vi "IDS Camera Engine.vi"(0 "IDS Notifier Name":string="Not a Name", 11 "Camera ID":string[](array[string])) -> ()   [LabVIEW 2020]
uses:
  IDS Controls/IDS Parameters.ctl
  IDS Controls/IDS Parameter List.ctl
  IDS Controls/IDS ROI.ctl
  IDS Controls/IDS Actions.ctl
  IDS Controls/IDS Notifier Element.ctl
  <vilib>/vision/Image Controls.llb/IMAQ Image.ctl
  C:/Users/Photonics03/Documents/Microscope-Control/Device Library/Cameras/IDS/IDS LabView Examples/LabVIEW/ueye.NET/uEyeDotNet.dll
  IDS LabView Examples/LabVIEW/ueye.NET/uEyeDotNet.dll
  Camera Controls/Camera IMAQ Key Info.ctl
panel:
  out "Image Key Error":errorcluster
  out "Frame":u32
  in  "Init Camera":bool
  in  "Quit":bool
  in  "Use Display Module":bool
  in  "Capture":bool
  in  "Live Preview":bool
  in  "Get ROI":bool
  in  "Set ROI":bool
  in  "Get Parameter":bool
  in  "Set Parameter":bool
  in  "File Save Path":path
  in  "# of Frames":u32
  in  "ROI Setup":T1
  in  "IDS Parameter":T2
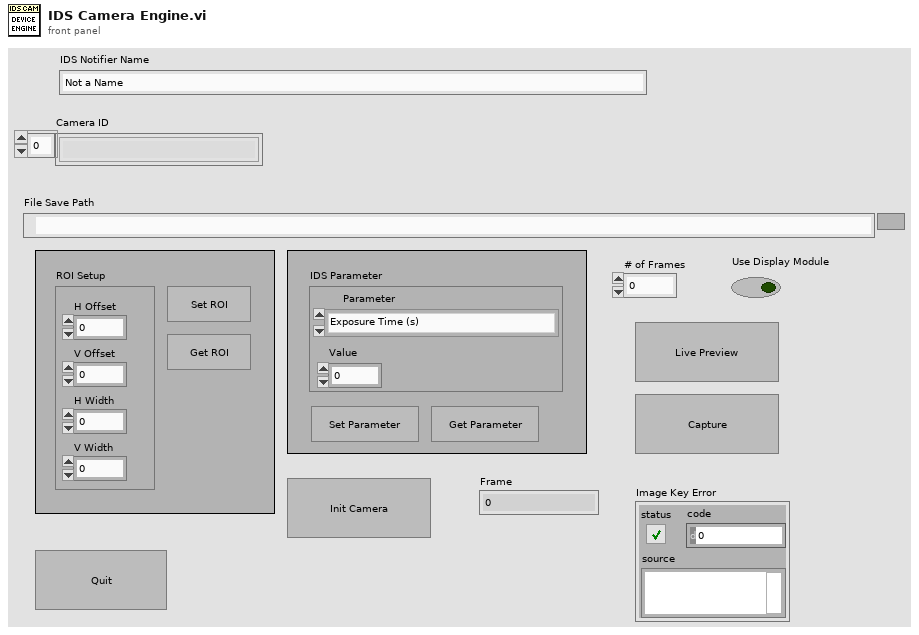
[diagram p1: front panel]
types:
  T1 = typedef "IDS ROI.ctl" = cluster{"H Offset":i32, "V Offset":i32, "H Width":i32, "V Width":i32}
  T2 = typedef "IDS Parameters.ctl" = cluster{"Parameter":T3, "Value":dbl}
  T3 = typedef "IDS Parameter List.ctl" = enum16{"Exposure Time (s)", "Binning"}
  T4 = typedef "IDS Notifier Element.ctl" = cluster{"IDS Actions":T5, "Received?":bool, "IDS Parameter":T2, "IDS ROI":T1, "Running?":bool, "File Path":path, "# of frames":u32, "Image Ref":T6, "Error":errorcluster, "Binning":i32}
  T5 = typedef "IDS Actions.ctl" = enum16{"Error Check", "Initialize", "Preview", "Record", "Abort", "Record Settings", "Set Parameter", "Get Parameter", "Set ROI", "Get ROI", "Status", "Quit"}
  T6 = typedef "IMAQ Image.ctl" = refnum<image>
  T7 = typedef "Image Type" = u32
  T8 = typedef "Camera IMAQ Key Info.ctl" = cluster{"Frame":u32, "Sensor Height":i32, "Sensor Width":i32, "ROI Height":i32, "ROI Width":i32, "ROI Enable?":bool, "Bit per Pixel":u8}
  T9 = enum32{"Invalid", "Standard", "Closed", "Hidden", "Minimized", "Maximized"}
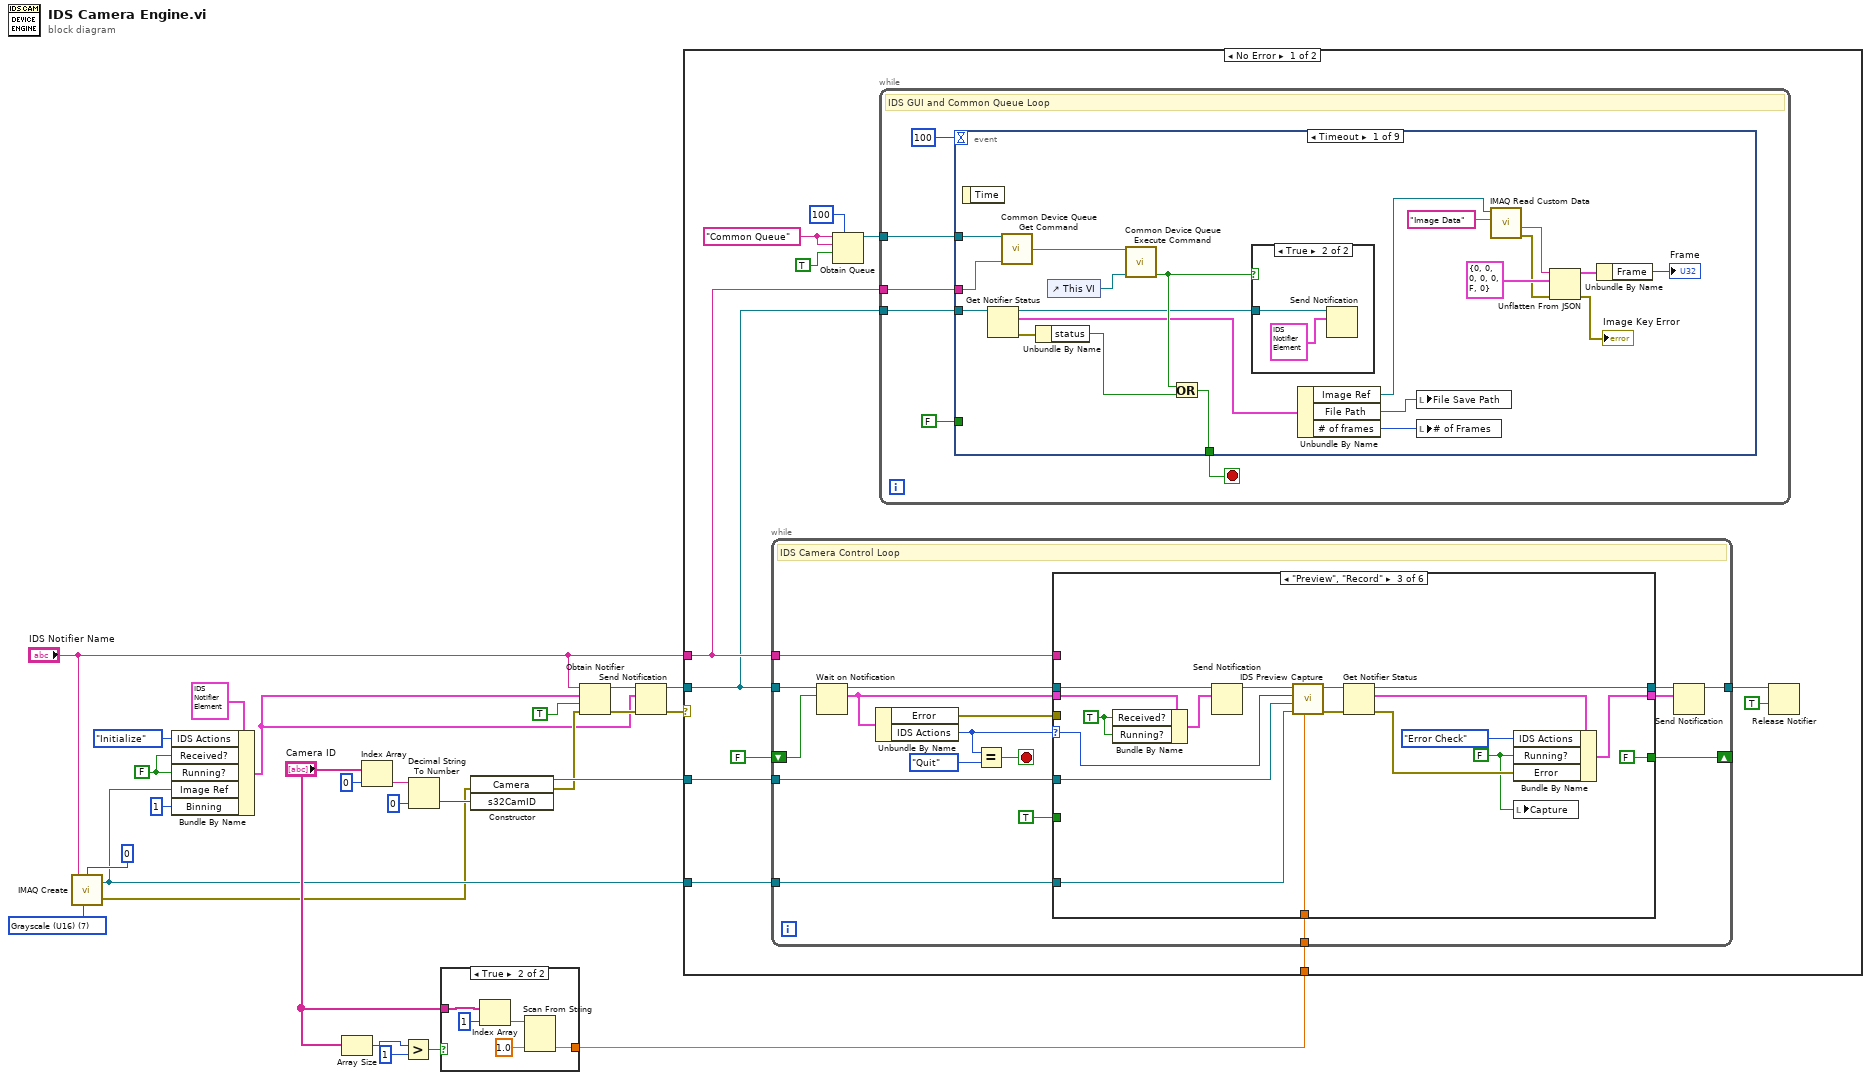
[diagram p0: block diagram]
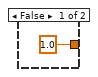
[diagram p2: hidden frame]
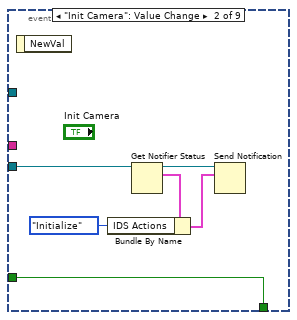
[diagram p4: hidden frame]
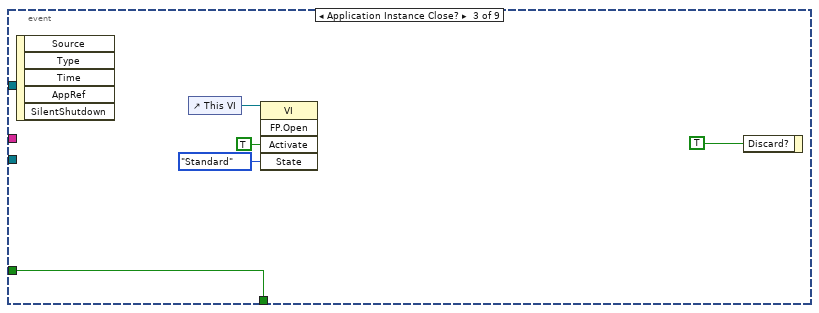
[diagram p5: hidden frame]
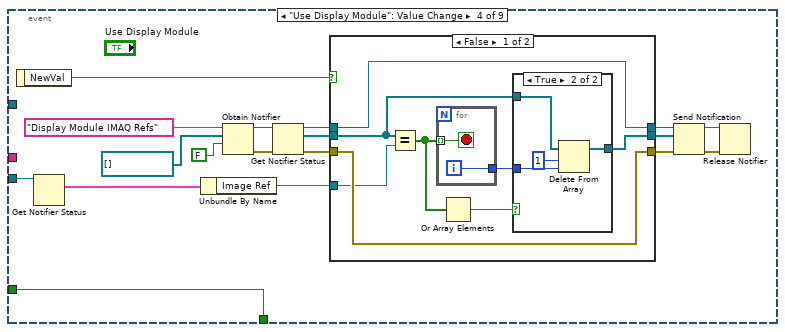
[diagram p6: hidden frame]
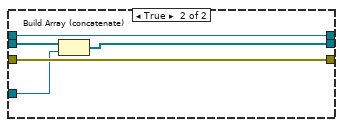
[diagram p8: hidden frame]
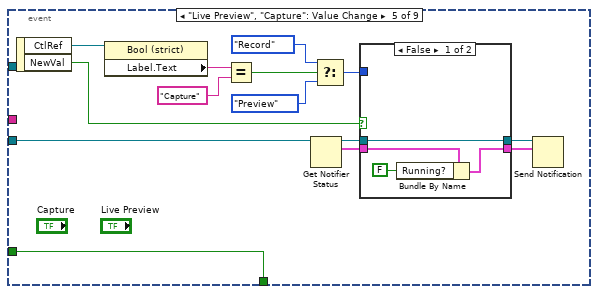
[diagram p9: hidden frame]
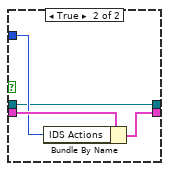
[diagram p10: hidden frame]
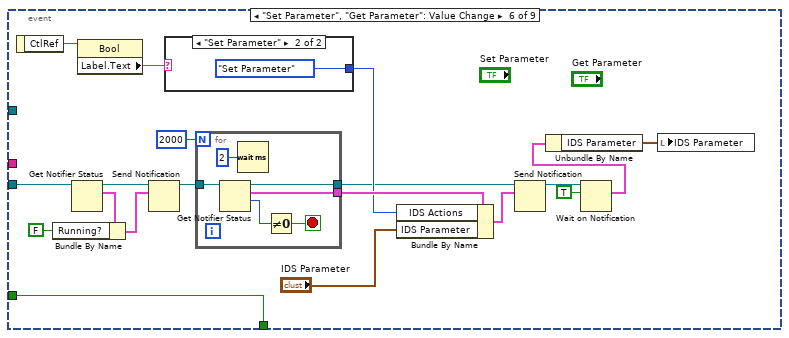
[diagram p11: hidden frame]
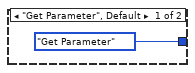
[diagram p12: hidden frame]
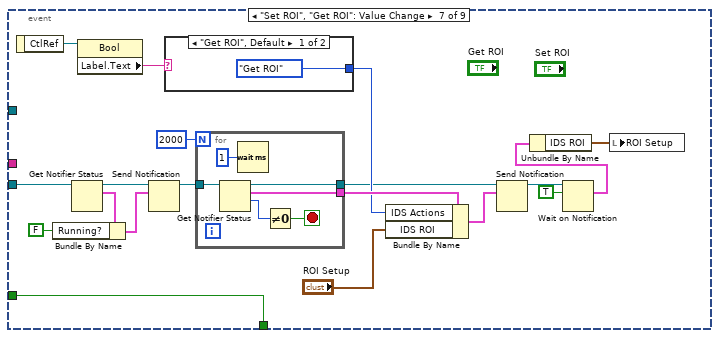
[diagram p13: hidden frame]
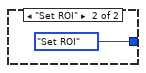
[diagram p14: hidden frame]
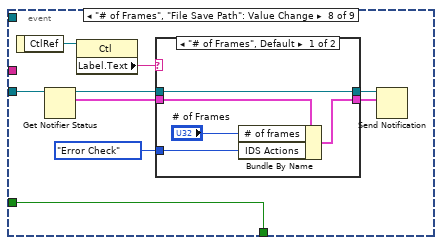
[diagram p15: hidden frame]
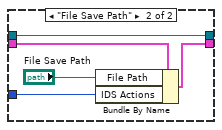
[diagram p16: hidden frame]
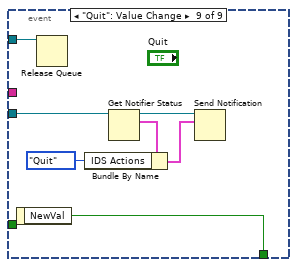
[diagram p17: hidden frame]
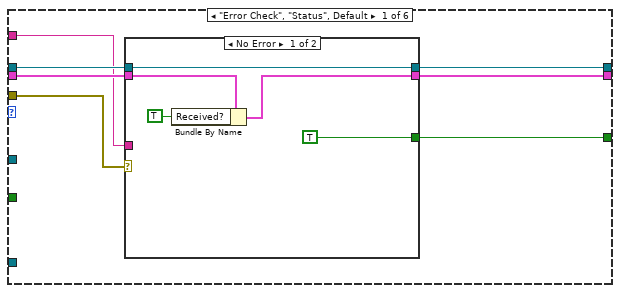
[diagram p18: hidden frame]
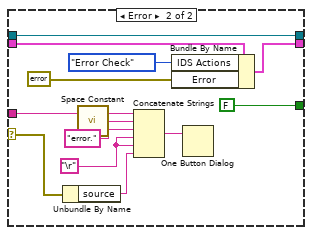
[diagram p19: hidden frame]
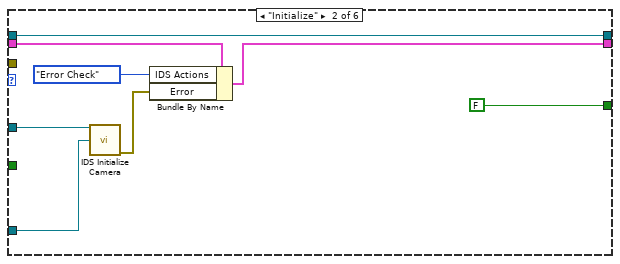
[diagram p20: hidden frame]
diagram:
  w2 = FALSE ("Received?")
  w16 = T7 7 items=["Grayscale (U8)", "Grayscale (I16)", "Grayscale (SGL)", "Complex (CSG)", "RGB (U32)", "HSL (U32)", "RGB (U64)", "Grayscale (U16)"] ("Image Type")
  n1 = call "IMAQ Create"("Border Size"=0, "Image Name"="IDS Notifier Name", "Image Type"=w16) -> ("New Image"=w14:T6, "error out"=w6:errorcluster)  [unwired: 2 in]
  n2 = Bundle By Name(cluster=T4 {"IDS Actions"=enum."Initialize", "Received?"=FALSE, "IDS Parameter"={"Parameter"=enum."Exposure Time (s)", "Value"=0.0}, "IDS ROI"={"H Offset"=0, "V Offset"=0, "H Width"=0, "V Width"=0}, "Running?"=FALSE, "File Path"=path "", "# of frames"=0, "Image Ref"=refnum, "Error"={"status"=FALSE, "code"=0, "source"=""}, "Binning"=0} ("IDS Camera Cluster"), "IDS Actions"=IDS_Actions."Initialize", "Received?"=w2, "Running?"=w2, "Image Ref"=w14, "Binning"=1) -> (w5:T4)
  n3 = Array Size(array="Camera ID") -> (size(s)=w12:i32)
  n4 = Index Array(array="Camera ID", index=0) -> (element=w19:string)
  n5 = Greater?(x=w12, y=1) -> (0:w11:bool)
  n6 = Decimal String To Number(string=w19, default (0L)=0 ("default (0 I32)")) -> (number=w7:i32)  [unwired: 1 in, 1 out]
  n7 = case shown="True" w11 {
    tunnel: "Camera ID" -> [_ w30]
    tunnel: [1.0 ("default (0 dbl)") w32] -> w13
    frame False {
    }
    frame True {
      n8 = Index Array(array=w30, index=1) -> (element=w31:string)
      n9 = Scan From String(input string=w31, default 1=1.0 ("default (0 dbl)")) -> (output 1=w32:dbl)  [unwired: 3 in, 3 out]
    }
  }
  n10 = constructor class="Camera"(error in=w6, "s32CamID"=w7) -> (reference out=w9:refnum<k24>, error out=w8:errorcluster)  [unwired: 2 in, 2 out]
  n11 = Obtain Notifier(name (unnamed)="IDS Notifier Name", notification data type=w5, create if not found? (T)=TRUE, error in (no error)=w8) -> (notifier out=w25:refnum<notifier>, error out=w24:errorcluster)  [unwired: 1 out]
  n12 = Send Notification(notification=w5, notifier=w25, error in (no error)=w24) -> (notifier out=w23:refnum<notifier>, error out=w22:errorcluster)
  n13 = case shown="No Error" w22 {
    selector: w22 -> [_ w341]
    tunnel: w23 -> [w34 w342]
    tunnel: "IDS Notifier Name" -> [w35 w340]
    tunnel: w9 -> [w42 w333]
    tunnel: w14 -> [w41 w332]
    tunnel: w13 -> [w33 _]
    frame No Error {
      w39 = "Common Queue" ("Unique Notifier Name")
      n14 = while {
        tunnel: w34 -> [w239]
        tunnel: [w240] -> w43
        tunnel: w42 -> [w233]
        tunnel: w41 -> [w232]
        shift-right: [w229] -> _
        shift-left: FALSE -> [w231]
        tunnel: w35 -> [w227]
        tunnel: w33 -> [w225]
        stop <- w241 stop-if-true
        # "IDS Camera Control Loop"
        n15 = Wait on Notification(notifier=w239, ignore previous (F)=w231) -> (notifier out=w238:refnum<notifier>, notification=w237:T4)  [unwired: 2 in, 2 out]
        n16 = Unbundle By Name(w237) -> ("Error"=w226:errorcluster, "IDS Actions"=w236:T5)
        n17 = Equal?(x=w236, y=IDS_Actions."Quit") -> (x = y?=w241:bool)
        n18 = case shown="\"Preview\", \"Record\"" w236 {
          selector: w236 -> [_ _ w277 w298 w312 _]
          tunnel: w238 -> [w247 w274 w292 w294 w315 w327]
          tunnel: [w246 w274 w289 w303 w306 w327] -> w234
          tunnel: w237 -> [w245 w272 w291 _ _ w325]
          tunnel: w227 -> [w244 _ _ _ _ _]
          tunnel: w233 -> [_ w273 w278 w297 w314 w321]
          tunnel: w232 -> [_ w267 w279 _ w313 w319]
          tunnel: [w243 w269 w288 w299 w305 w323] -> w230
          tunnel: [w248 FALSE FALSE FALSE w316 w326] -> w229
          tunnel: TRUE -> [_ _ _ _ w316 w326]
          tunnel: w226 -> [w242 _ _ w296 _ w317]
          tunnel: w225 -> [_ _ w275 _ _ _]
          frame "Error Check", "Status", Default {
            n19 = case shown="No Error" w242 {
              selector: w242 -> [_ w256]
              tunnel: w245 -> [w251 w266]
              tunnel: [TRUE FALSE] -> w248
              tunnel: [w253 w263] -> w246
              tunnel: w247 -> [w253 w263]
              tunnel: w244 -> [_ w262]
              tunnel: [w249 w258] -> w243
              frame No Error {
                n20 = Bundle By Name(cluster=w251, "Received?"=TRUE) -> (w249:T4)
              }
              frame Error {
                w257 = "\r"
                n21 = Unbundle By Name(w256) -> ("source"=w255:string)
                n22 = call <vilib>:"Space Constant.vi"() -> ("String"=w261:string)
                n23 = Concatenate Strings(w262, w261, "error." ("string"), w257, w257, w255) -> (w259:string)
                n24 = Bundle By Name(cluster=w266, "IDS Actions"=IDS_Actions."Error Check", "Error"=errorcluster {"status"=FALSE, "code"=0, "source"=""}) -> (w258:T4)
                n25 = One Button Dialog(message=w259) -> ()  [unwired: 1 in, 1 out]
              }
            }
          }
          frame "Initialize" {
            n26 = call "IDS Initialize Camera.vi"("Camera ID"=w273, "IDS Cam Img Ref"=w267) -> ("Error Out"=w270:errorcluster)  [unwired: 12 in, 1 out]
            n27 = Bundle By Name(cluster=w272, "IDS Actions"=IDS_Actions."Error Check", "Error"=w270) -> (w269:T4)
          }
          frame "Preview", "Record" {
            w276 = FALSE ("Running?")
            w285 = TRUE ("Received?")
            n28 = Bundle By Name(cluster=w291, "Received?"=w285, "Running?"=w285) -> (w287:T4)
            n29 = Send Notification(notification=w287, notifier=w292) -> (notifier out=w284:refnum<notifier>)  [unwired: 1 in, 1 out]
            n30 = call "IDS Preview Capture.vi"("Pixel Size (µm)"=w275, "Image Ref"=w279, "IDS Camera Ref"=w278, "IDS Actions"=w277, "IDS Notifier"=w284) -> ("Error"=w281:errorcluster, "IDS Notifier"=w283:refnum<notifier>)  [unwired: 5 in]
            n31 = Get Notifier Status(notifier=w283, error in (no error)=w281) -> (notifier out=w289:refnum<notifier>, current notification=w282:T4, error out=w280:errorcluster)  [unwired: 2 out]
            n32 = Bundle By Name(cluster=w282, "IDS Actions"=IDS_Actions."Error Check", "Running?"=w276, "Error"=w280) -> (w288:T4)
            n33 = local write "Capture"(w276) -> ()
          }
          frame "Set Parameter", "Get Parameter" {
            n34 = call "IDS Set Get Parameter.vi"("IDS Notifier"=w294, "IDS Actions"=w298, "IDS Camera Ref"=w297, "Error"=w296) -> ("IDS Notifier"=w304:refnum<notifier>, "Error"=w300:errorcluster)  [unwired: 10 in]
            n35 = Get Notifier Status(notifier=w304) -> (notifier out=w303:refnum<notifier>, current notification=w302:T4)  [unwired: 1 in, 3 out]
            n36 = Bundle By Name(cluster=w302, "IDS Actions"=IDS_Actions."Error Check", "Error"=w300, "Received?"=TRUE) -> (w299:T4)
          }
          frame "Set ROI", "Get ROI" {
            n37 = call "IDS Set Get ROI.vi"("IDS Notifier Ref"=w315, "IDS Actions"=w312, "IDS Camera Ref"=w314, "IDS Image Ref"=w313) -> ("IDS Notifier Ref (Dup)"=w307:refnum<notifier>, "Error"=w308:errorcluster)  [unwired: 10 in]
            n38 = Get Notifier Status(notifier=w307) -> (notifier out=w306:refnum<notifier>, current notification=w311:T4)  [unwired: 1 in, 3 out]
            n39 = Bundle By Name(cluster=w311, "IDS Actions"=IDS_Actions."Error Check", "Error"=w308, "Received?"=TRUE) -> (w305:T4)
          }
          frame "Quit" {
            n40 = call "IMAQ Dispose"("Image"=w319) -> ()  [unwired: 5 in, 1 out]
            n41 = invoke class="Camera" method="Exit"(reference=w321, error in=w317) -> (reference out=w322:refnum<k24>, error out=w320:errorcluster)  [unwired: 1 in, 1 out]
            n42 = Close Reference(reference=w322, error in (no error)=w320) -> (error out=w318:errorcluster)
            n43 = Bundle By Name(cluster=w325, "Received?"=TRUE, "Error"=w318) -> (w323:T4)
          }
        }
        n44 = Send Notification(notification=w230, notifier=w234) -> (notifier out=w240:refnum<notifier>)  [unwired: 1 in, 1 out]
      }
      n45 = Obtain Queue(max queue size (-1, unlimited)=100, name (unnamed)=w39, element data type=w39, create if not found? (T)=TRUE) -> (queue out=w36:refnum<queue>)  [unwired: 1 in, 2 out]
      n46 = while {
        tunnel: w36 -> [w49]
        tunnel: w35 -> [w47]
        tunnel: w34 -> [w48]
        stop <- w46 stop-if-true
        # "IDS GUI and Common Queue Loop"
        n47 = event shown="[0] Timeout" {
          selector: _ -> [_ _ _ _ _ _ _ _ _]
          dyn-events: _ -> [_ _ _ _ _ _ _ _ _]
          timeout: 100 -> [_ _ _ _ _ _ _ _ _]
          tunnel: w49 -> [w65 _ _ _ _ _ _ _ w224]
          tunnel: w48 -> [w64 w78 _ w102 w127 w161 w188 w205 w223]
          tunnel: w47 -> [w63 _ _ _ _ _ _ _ _]
          tunnel: [w62 w79 w84 w85 w136 w163 w190 w207 w218] -> w46
          tunnel: FALSE -> [_ w79 w84 w85 w136 w163 w190 w207 _]
          event Timeout {
            n48 = event-data() -> ()  [unwired: 1 in, 1 out]
            n49 = Get Notifier Status(notifier=w64) -> (notifier out=w66:refnum<notifier>, current notification=w59:T4, error out=w71:errorcluster)  [unwired: 1 in, 2 out]
            n50 = call "Common Device Queue Get Command.vi"("Common Queue"=w65, "Notifier Name"=w63) -> ("Command"=w70:string)  [unwired: 12 in, 1 out]
            n51 = Unbundle By Name(w71) -> ("status"=w68:bool)
            n52 = control-ref of="This VI"() -> (w69:refnum<vi>)
            n53 = call "Common Device Queue Execute Command.vi"("Common Command"=w70, "VI Refnum"=w69) -> ("Quit?"=w67:bool)  [unwired: 12 in, 1 out]
            n54 = Or(x=w67, y=w68) -> (x .or. y?=w62:bool)
            n55 = case shown="True" w67 {
              tunnel: w66 -> [_ w73]
              frame False {
              }
              frame True {
                n56 = Send Notification(notification=T4 {"IDS Actions"=enum."Quit", "Received?"=FALSE, "IDS Parameter"={"Parameter"=enum."Exposure Time (s)", "Value"=0.0}, "IDS ROI"={"H Offset"=0, "V Offset"=0, "H Width"=0, "V Width"=0}, "Running?"=FALSE, "File Path"=path "", "# of frames"=0, "Image Ref"=refnum, "Error"={"status"=FALSE, "code"=0, "source"=""}, "Binning"=0} ("IDS Camera Cluster"), notifier=w73) -> ()  [unwired: 1 in, 2 out]
              }
            }
            n57 = Unbundle By Name(w59) -> ("Image Ref"=w57:T6, "File Path"=w61:path, "# of frames"=w60:u32)
            n58 = local write "File Save Path"(w61) -> ()
            n59 = local write "# of Frames"(w60) -> ()
            n60 = call "IMAQ Read Custom Data"("Key"="Image Data", "Image"=w57) -> ("error out"=w52:errorcluster, "Custom Data Out"=w55:string)  [unwired: 7 in, 1 out]
            n61 = Unflatten From JSON(JSON string=w55, type and defaults=T8 {"Frame"=0, "Sensor Height"=0, "Sensor Width"=0, "ROI Height"=0, "ROI Width"=0, "ROI Enable?"=FALSE, "Bit per Pixel"=0} ("Camera IMAQ Key Info"), error in (no error)=w52) -> (value=w54:T8, error out=→"Image Key Error":errorcluster)  [unwired: 4 in]
            n62 = Unbundle By Name(w54) -> ("Frame"=→"Frame":u32)
          }
          event "Init Camera": Value Change {
            n63 = event-data() -> ()  [unwired: 1 in, 1 out]
            n64 = Get Notifier Status(notifier=w78) -> (notifier out=w74:refnum<notifier>, current notification=w77:T4)  [unwired: 1 in, 3 out]
            n65 = Bundle By Name(cluster=w77, "IDS Actions"=IDS_Actions."Initialize") -> (w75:T4)
            n66 = Send Notification(notification=w75, notifier=w74) -> ()  [unwired: 1 in, 2 out]
          }
          event Application Instance Close? {
            n67 = event-data() -> ()  [unwired: 1 in, 5 out]
            n68 = control-ref of="This VI"() -> (w81:refnum<vi>)
            n69 = invoke class="VI" method="FP.Open"(reference=w81, "Activate"=TRUE ("Activate?"), "State"=T9."Standard") -> ()  [unwired: 2 in, 5 out]
            n70 = event-data("Discard?"=TRUE) -> ()  [unwired: 1 in, 1 out]
          }
          event "Use Display Module": Value Change {
            n71 = event-data() -> ("NewVal"=w87:bool)  [unwired: 1 in]
            n72 = Get Notifier Status(notifier=w102) -> (current notification=w101:T4)  [unwired: 1 in, 4 out]
            n73 = Unbundle By Name(w101) -> ("Image Ref"=w86:T6)
            n74 = Obtain Notifier(name (unnamed)="Display Module IMAQ Refs", notification data type=T6[] [], create if not found? (T)=FALSE) -> (notifier out=w94:refnum<notifier>, error out=w93:errorcluster)  [unwired: 1 in, 1 out]
            n75 = Get Notifier Status(notifier=w94, error in (no error)=w93) -> (notifier out=w95:refnum<notifier>, current notification=w97:T6[], error out=w96:errorcluster)  [unwired: 2 out]
            n76 = case shown="False" w87 {
              tunnel: w95 -> [w110 w120]
              tunnel: w96 -> [w104 w119]
              tunnel: w97 -> [w106 w122]
              tunnel: [w105 w121] -> w100
              tunnel: [w110 w120] -> w98
              tunnel: [w104 w119] -> w99
              tunnel: w86 -> [w103 w118]
              frame False {
                n77 = Equal?(x=w106, y=w103) -> (x = y?=w109:bool[])
                n78 = for {
                  tunnel: w109 -> [w117] mode=indexing
                  tunnel: [w116] -> w107
                  i -> [w116]
                  stop <- w117 stop-if-true
                }
                n79 = Or Array Elements(Boolean array=w109) -> (logical OR=w108:bool)
                n80 = case shown="True" w108 {
                  tunnel: w107 -> [_ w114]
                  tunnel: w106 -> [w111 w113]
                  tunnel: [w111 w112] -> w105
                  frame False {
                  }
                  frame True {
                    n81 = Delete From Array(array=w113, length=1, index=w114) -> (array with subset deleted=w112:T6[])  [unwired: 1 out]
                  }
                }
              }
              frame True {
                n82 = Build Array (concatenate)(w122, w118) -> (w121:T6[])
              }
            }
            n83 = Send Notification(notification=w100, notifier=w98, error in (no error)=w99) -> (notifier out=w92:refnum<notifier>, error out=w91:errorcluster)
            n84 = Release Notifier(notifier=w92, error in (no error)=w91) -> ()  [unwired: 1 in, 3 out]
          }
          event "Live Preview", "Capture": Value Change {
            n85 = event-data() -> ("CtlRef"=w135:refnum<vi>, "NewVal"=w129:bool)  [unwired: 1 in]
            n86 = property class="Bool (strict)"(reference=w135) -> ("Label.Text"=w134:string)  [unwired: 1 in, 2 out]
            n87 = Equal?(x=w134, y="Capture") -> (x = y?=w132:bool)
            n88 = Get Notifier Status(notifier=w127) -> (notifier out=w126:refnum<notifier>, current notification=w125:T4)  [unwired: 1 in, 3 out]
            n89 = Select(t=IDS_Actions."Record" ("y"), s=w132, f=IDS_Actions."Preview" ("y")) -> (s? t:f=w128:T5)
            n90 = case shown="False" w129 {
              tunnel: w128 -> [_ w143]
              tunnel: w126 -> [w138 w142]
              tunnel: w125 -> [w140 w144]
              tunnel: [w138 w142] -> w124
              tunnel: [w137 w141] -> w123
              frame False {
                n91 = Bundle By Name(cluster=w140, "Running?"=FALSE) -> (w137:T4)
              }
              frame True {
                n92 = Bundle By Name(cluster=w144, "IDS Actions"=w143) -> (w141:T4)
              }
            }
            n93 = Send Notification(notification=w123, notifier=w124) -> ()  [unwired: 1 in, 2 out]
          }
          event "Set Parameter", "Get Parameter": Value Change {
            n94 = event-data() -> ("CtlRef"=w162:refnum<vi>)  [unwired: 1 in]
            n95 = Get Notifier Status(notifier=w161) -> (notifier out=w156:refnum<notifier>, current notification=w159:T4)  [unwired: 1 in, 3 out]
            n96 = Bundle By Name(cluster=w159, "Running?"=FALSE) -> (w155:T4)
            n97 = property class="Bool"(reference=w162) -> ("Label.Text"=w160:string)  [unwired: 1 in, 2 out]
            n98 = Send Notification(notification=w155, notifier=w156) -> (notifier out=w154:refnum<notifier>)  [unwired: 1 in, 1 out]
            n99 = case shown="\"Set Parameter\"" w160 {
              tunnel: [IDS_Actions."Get Parameter" ("IDS Actions") IDS_Actions."Set Parameter" ("IDS Actions")] -> w151
              frame "Get Parameter", Default {
              }
              frame "Set Parameter" {
              }
            }
            n100 = for {
              N: 2000 -> [_]
              tunnel: w154 -> [w168]
              tunnel: [w167] -> w150
              tunnel: [w166] -> w153
              stop <- w164 stop-if-true
              n101 = Get Notifier Status(notifier=w168) -> (notifier out=w167:refnum<notifier>, current notification=w166:T4, # waiting=w165:i32)  [unwired: 1 in, 2 out]
              n102 = Wait (ms)(milliseconds to wait=u32 2) -> ()  [unwired: 1 out]
              n103 = Not Equal To 0?(x=w165) -> (x != 0?=w164:bool)
            }
            n104 = Bundle By Name(cluster=w153, "IDS Actions"=w151, "IDS Parameter"="IDS Parameter") -> (w149:T4)
            n105 = Send Notification(notification=w149, notifier=w150) -> (notifier out=w148:refnum<notifier>)  [unwired: 1 in, 1 out]
            n106 = Wait on Notification(notifier=w148, ignore previous (F)=TRUE) -> (notification=w146:T4)  [unwired: 2 in, 3 out]
            n107 = Unbundle By Name(w146) -> ("IDS Parameter"=w145:T2)
            n108 = local write "IDS Parameter"(w145) -> ()
          }
          event "Set ROI", "Get ROI": Value Change {
            n109 = event-data() -> ("CtlRef"=w189:refnum<vi>)  [unwired: 1 in]
            n110 = Get Notifier Status(notifier=w188) -> (notifier out=w183:refnum<notifier>, current notification=w186:T4)  [unwired: 1 in, 3 out]
            n111 = Bundle By Name(cluster=w186, "Running?"=FALSE) -> (w182:T4)
            n112 = property class="Bool"(reference=w189) -> ("Label.Text"=w187:string)  [unwired: 1 in, 2 out]
            n113 = Send Notification(notification=w182, notifier=w183) -> (notifier out=w181:refnum<notifier>)  [unwired: 1 in, 1 out]
            n114 = case shown="\"Get ROI\", Default" w187 {
              tunnel: [IDS_Actions."Get ROI" ("IDS Actions") IDS_Actions."Set ROI" ("IDS Actions")] -> w179
              frame "Get ROI", Default {
              }
              frame "Set ROI" {
              }
            }
            n115 = for {
              N: 2000 -> [_]
              tunnel: w181 -> [w195]
              tunnel: [w194] -> w178
              tunnel: [w193] -> w180
              stop <- w191 stop-if-true
              n116 = Get Notifier Status(notifier=w195) -> (notifier out=w194:refnum<notifier>, current notification=w193:T4, # waiting=w192:i32)  [unwired: 1 in, 2 out]
              n117 = Wait (ms)(milliseconds to wait=u32 1) -> ()  [unwired: 1 out]
              n118 = Not Equal To 0?(x=w192) -> (x != 0?=w191:bool)
            }
            n119 = Bundle By Name(cluster=w180, "IDS Actions"=w179, "IDS ROI"="ROI Setup") -> (w177:T4)
            n120 = Send Notification(notification=w177, notifier=w178) -> (notifier out=w176:refnum<notifier>)  [unwired: 1 in, 1 out]
            n121 = Wait on Notification(notifier=w176, ignore previous (F)=TRUE) -> (notification=w174:T4)  [unwired: 2 in, 3 out]
            n122 = Unbundle By Name(w174) -> ("IDS ROI"=w173:T1)
            n123 = local write "ROI Setup"(w173) -> ()
          }
          event "# of Frames", "File Save Path": Value Change {
            n124 = event-data() -> ("CtlRef"=w206:refnum<vi>)  [unwired: 1 in]
            n125 = Get Notifier Status(notifier=w205) -> (notifier out=w203:refnum<notifier>, current notification=w202:T4)  [unwired: 1 in, 3 out]
            n126 = property class="Ctl"(reference=w206) -> ("Label.Text"=w204:string)  [unwired: 1 in, 2 out]
            n127 = case shown="\"# of Frames\", Default" w204 {
              tunnel: w203 -> [w210 w217]
              tunnel: w202 -> [w212 w216]
              tunnel: [w210 w217] -> w201
              tunnel: [w209 w215] -> w200
              tunnel: IDS_Actions."Error Check" ("IDS Actions") -> [w208 w213]
              frame "# of Frames", Default {
                n128 = Bundle By Name(cluster=w212, "# of frames"="# of Frames", "IDS Actions"=w208) -> (w209:T4)
              }
              frame "File Save Path" {
                n129 = Bundle By Name(cluster=w216, "File Path"="File Save Path", "IDS Actions"=w213) -> (w215:T4)
              }
            }
            n130 = Send Notification(notification=w200, notifier=w201) -> ()  [unwired: 1 in, 2 out]
          }
          event "Quit": Value Change {
            n131 = event-data() -> ("NewVal"=w218:bool)  [unwired: 1 in]
            n132 = Release Queue(queue=w224) -> ()  [unwired: 2 in, 3 out]
            n133 = Get Notifier Status(notifier=w223) -> (notifier out=w222:refnum<notifier>, current notification=w221:T4)  [unwired: 1 in, 3 out]
            n134 = Bundle By Name(cluster=w221, "IDS Actions"=IDS_Actions."Quit") -> (w219:T4)
            n135 = Send Notification(notification=w219, notifier=w222) -> ()  [unwired: 1 in, 2 out]
          }
        }
      }
      n136 = Release Notifier(notifier=w43, force destroy? (F)=TRUE) -> ()  [unwired: 1 in, 3 out]
    }
    frame Error {
      n137 = Release Notifier(notifier=w342, force destroy? (F)=TRUE, error in (no error)=w341) -> (error out=w331:errorcluster)  [unwired: 2 out]
      n138 = invoke class="Camera" method="Exit"(reference=w333, error in=w331) -> (reference out=w334:refnum<k24>, error out=w330:errorcluster)  [unwired: 1 in, 1 out]
      n139 = Close Reference(reference=w334, error in (no error)=w330) -> (error out=w329:errorcluster)
      n140 = call "IMAQ Dispose"("Image"=w332, "error in (no error)"=w329) -> ("error out"=w328:errorcluster)  [unwired: 4 in]
      n141 = Unbundle By Name(w328) -> ("source"=w335:string)
      n142 = call <vilib>:"Space Constant.vi"() -> ("String"=w338:string)
      n143 = Concatenate Strings(w340, w338, "Device Error." ("string"), "\r", w335) -> (w339:string)
      n144 = One Button Dialog(message=w339) -> ()  [unwired: 1 in, 1 out]
    }
  }
